vi "5p1_HW_Task2_pipoat.vi"() -> ()   [LabVIEW 2016]
panel:
  out "Test Result":string
  in  "F''(x)":dbl
  in  "F'(x)":dbl
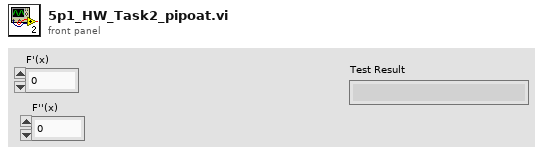
[diagram p1: front panel]
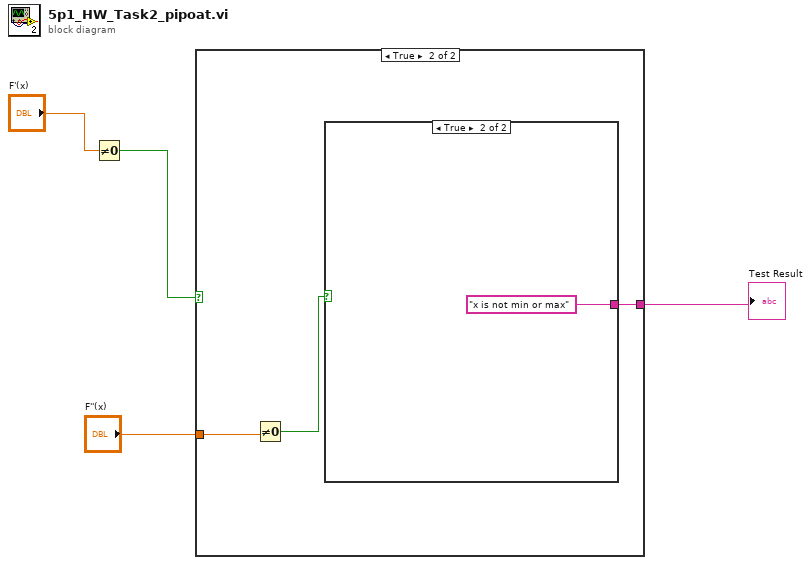
[diagram p0: block diagram]
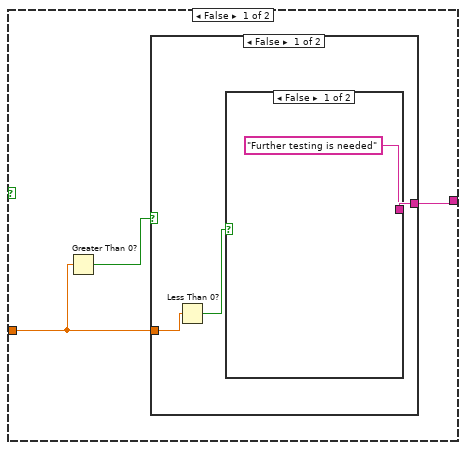
[diagram p2: hidden frame]
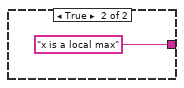
[diagram p3: hidden frame]
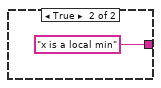
[diagram p4: hidden frame]
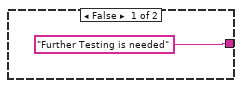
[diagram p5: hidden frame]
diagram:
  n1 = Not Equal To 0?(x="F'(x)") -> (x != 0?=w3:bool)
  n2 = case shown="True" w3 {
    tunnel: "F''(x)" -> [w5 w16]
    tunnel: [w6 w14] -> w1
    frame False {
      n3 = Greater Than 0?(x=w5) -> (x > 0?=w7:bool)
      n4 = case shown="False" w7 {
        tunnel: [w8 "x is a local min"] -> w6
        tunnel: w5 -> [w10 _]
        frame False {
          n5 = Less Than 0?(x=w10) -> (x < 0?=w9:bool)
          n6 = case shown="False" w9 {
            tunnel: ["Further testing is needed" "x is a local max"] -> w8
            frame False {
            }
            frame True {
            }
          }
        }
        frame True {
        }
      }
    }
    frame True {
      n7 = Not Equal To 0?(x=w16) -> (x != 0?=w15:bool)
      n8 = case shown="True" w15 {
        tunnel: ["Further Testing is needed" "x is not min or max"] -> w14
        frame False {
        }
        frame True {
        }
      }
    }
  }
  "Test Result" <- w1
